vi "user32_SetWindowLongA.vi"(8 "error in (no error)":errorcluster, 9 "dwNewLong":i32, 10 "nIndex":i32, 11 "hWnd":i64) -> (0 "error out":errorcluster, 3 "return":i64)   [LabVIEW 2020]
uses:
  user32.dll
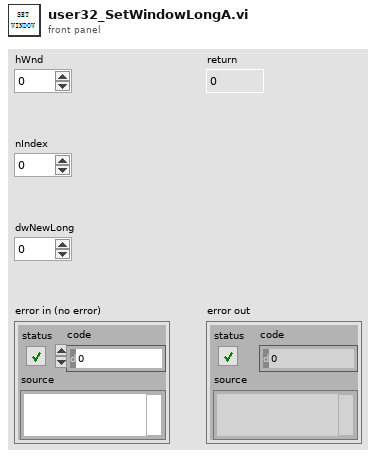
[diagram p1: front panel]
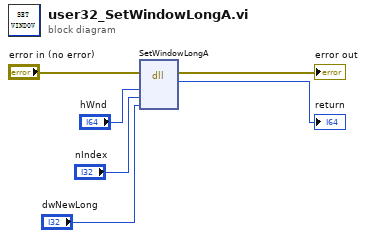
[diagram p0: block diagram]
diagram:
  n1 = dll-call lib="user32.dll" fn="SetWindowLongA"(error in="error in (no error)", "hWnd"="hWnd", "nIndex"="nIndex", "dwNewLong"="dwNewLong") -> (error out=→"error out":errorcluster, "返回值"=→"return":i64)  [unwired: 5 in, 1 out]
